vi "Disable And Grey Out GUI Objects.vi"(8 "Error In":errorcluster, 11 "GUI Object Refs":refnum<vi>[](array[refnum])) -> (0 "Error Out":errorcluster)   [LabVIEW 2022 SP3]
doc: "Disables and greys out GUI Objects"
panel:
  # "Development\nControls or indicators that are useful for development or testing, but which are not outputs of the VI."
  # "Input\nInputs to the VI"
  # "Output\nOutputs of the VI"
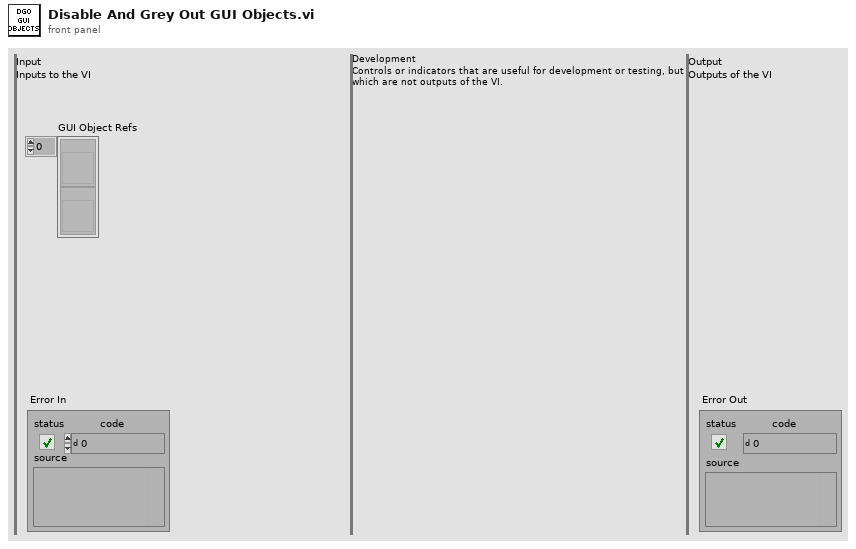
[diagram p1: front panel]
types:
  T1 = enum8{"Enabled", "Disabled", "Disabled and Grayed Out"}
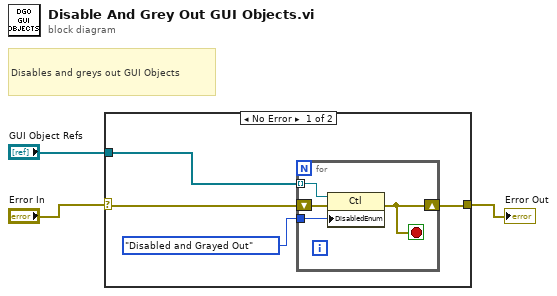
[diagram p0: block diagram]
diagram:
  # "Disables and greys out GUI Objects"
  n1 = case shown="No Error" "Error In" {
    selector: "Error In" -> [w6 w12]
    tunnel: [w5 w12] -> w2
    tunnel: "GUI Object Refs" -> [w4 _]
    frame No Error {
      n2 = for {
        shift-right: [w8] -> w5
        shift-left: w6 -> [w11]
        tunnel: w4 -> [w10] mode=indexing
        tunnel: T1."Disabled and Grayed Out" ("Disabled") -> [w9]
        stop <- w8 stop-if-true
        n3 = property class="Ctl"(reference=w10, error in=w11, "DisabledEnum"=w9) -> (error out=w8:errorcluster)  [unwired: 1 out]
      }
    }
    frame Error {
    }
  }
  "Error Out" <- w2
